vi "Read Chip.vi"(1 "Config Bits":T1[](array[typedef])=[8, 0, 0, 0, 0, 0, 0, 0] items=["Ch 0 SE"=8, "Ch 1 SE"=9, "Ch 2 SE"=10, "Ch 3 SE"=11, "Ch 4 SE"=12, "Ch 5 SE"=13, "Ch 6 SE"=14, "Ch 7 SE"=15, "Diff 0+ 1-"=0, "Diff 1+ 0-"=1, "Diff 2+ 3-"=2, "Diff 3+ 2-"=3, "Diff 4+ 5-"=4, "Diff 5+ 4-"=5, "Diff 6+ 7-"=6, "Diff 7+ 6-"=7], 2 "ADC CS line":refnum<k21>="AI_CS1") -> (0 "Read Values":u16[](array[numeric]))   [LabVIEW 2018, in "MCP3008.lvlib"]
uses:
  MCP3008.lvlib
  Configuration Bits.ctl
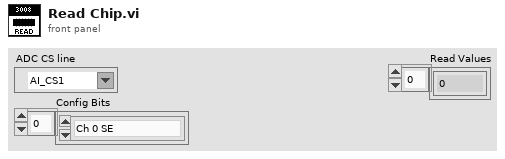
[diagram p1: front panel]
types:
  T1 = typedef "MCP3008.lvlib/Configuration Bits.ctl" = u8
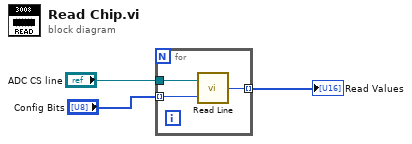
[diagram p0: block diagram]
diagram:
  n1 = for {
    tunnel: "ADC CS line" -> [w6]
    tunnel: "Config Bits" -> [w5] mode=indexing
    tunnel: [w4] -> w2 mode=indexing
    n2 = call "Read Line.vi"("Configuration Bits"=w5, "ADC CS line"=w6) -> ("number"=w4:u16)
  }
  "Read Values" <- w2
